vi "Dashboard Main.vi"() -> ()   [LabVIEW 2015]
uses:
  <vilib>/Rock Robotics/WPI/DriverStation/WPI_DriverStationRobotMode2.ctl
  <vilib>/event_ctls.llb/eventvkey.ctl
  <vilib>/Rock Robotics/WPI/Dashboard/WPI_DashboardLogging Global.vi
  <vilib>/Rock Robotics/Network Tables/NT Read Numeric Array.vi
  <vilib>/Rock Robotics/Network Tables/SD Read Number.vi
  <vilib>/Rock Robotics/Network Tables/SD Write Number.vi
  <vilib>/Rock Robotics/Network Tables/SD Write Boolean.vi
  <vilib>/Rock Robotics/Network Tables/SD Read Boolean.vi
  <vilib>/Rock Robotics/Network Tables/NT Write Boolean.vi
  <vilib>/Utility/config.llb/Write Key (String).vi
  <vilib>/Utility/config.llb/Write Key (I32).vi
  <vilib>/Utility/config.llb/NI_LVConfig.lvlib
panel:
  out "x = 0?":bool[](array[boolean])
  in  "TCP":refnum<k5>
  out "Camera IP":string
  out "Image Message":string="Timeout in Camera Communications"
  in  "Dashboard Tab":T1(tab)
  in  "Force Aim":bool
  in  "Enable Shooter":bool=TRUE
  in  "Intake to top?":bool=TRUE
  in  "Straight Forward":bool
  in  "Camera Settings":T2={"Frame Rate"=30, "Compression"=30, "Size"=1} {"Frame Rate" scale=1.0..30.0; "Size" items=["640x480", "320x240", "160x120"]}
  out "MotorChart R":cluster{"Numeric":dbl, "Numeric":dbl}(graph)
  out "MotorChart L":T3(graph)
  out "MotorSliders R":cluster{"MotorSlide1":dbl, "MotorSlide2":dbl} {"MotorSlide2" scale=-1.0..1.0 scale format="%#_2e"; "MotorSlide1" scale=-1.0..1.0 scale format="%#_2e"}
  out "MotorSliders L":T4 {"MotorSlide4 2" scale=0.0..14.0 scale format="%#_2e"; "MotorSlide2" scale=-1.0..1.0 scale format="%#_2e"; "MotorSlide1" scale=-1.0..1.0 scale format="%#_2e"}
  out "Yaw":dbl(knob) scale=180.0..-180.0
  out "JS1 Z":dbl(slide) scale=-1.0..1.0 scale format="%#_2e"
  out "JS1 Graph":cluster{"X":dbl, "Y":dbl}[](graph)
  out "JS1 Buttons":T5
  out "JS2 Z":dbl(slide) scale=-1.0..1.0 scale format="%#_2e"
  out "JS2 Graph":cluster{"X":dbl, "Y":dbl}[](graph)
  out "JS2 Buttons":T5
  out "Mode":T6(ring)=enum."Auto Disabled"
  in  "DB Camera Config":bool
  out "fps":dbl format="%#.1g"
  out "Mbps":dbl format="%#.1g"
  out "Mbps 2":bool
  out "Goal Detected":bool
  out "Ball Detected":bool
  in  "Start with Ball?":bool
  in  "Drive speed (0-1)":dbl
  in  "In. to Drive":dbl
  in  "Start Position":T7(ring)
  in  "Drive Back?":bool
  in  "Auto Mode":T8(ring)
  in  "Turn Around?":bool
  out "CAN Errors":T9(graph)
  out "Drive":T9(graph)
  out "Current":T9(graph)
  out "Drive Throttle":T9(graph)
  out "?":T10(graph)
  out "?":T9(graph)
  out "?":T10(graph)
  out "?":T10(graph)
  out "?":T9(graph)
  out "?":T10(graph)
  out "?":T9(graph)
  out "?":T9(graph)
  in  "Test Slider":dbl(slide) scale=0.0..100.0 scale format="%#_3g"
  in  "On/Off":bool caption="Solenoid"
  in  "Test Name":u16(ring) items=["Select the test to run...", "Example Test", "-------------------------------", "List of tests is built in robot code.", "Replace with your own automated tests."]
  in  "Test Tree":string(tree)
  in  "Motor":cluster{"Value":dbl, "Enable":bool} {"Value" scale=-1.0..1.0 scale format="%#_3g"}
  out "Progress":T11 {"Test Progress" scale=0.0..100.0}
  in  "Rev/Fwd":cluster{"Forward":bool, "Reverse":bool}
  in  "Test Ring":u16(ring) items=["Monochrome", "Color"]
  in  "Vision":u16(ring) items=["Camera Off", "USB Camera SW", "USB Camera HW", "IP Camera"]
  in  "Rec Mode":enum32{"Stop", "Record", "Playback"}(radio)
  in  "Listbox":i32(listbox)
  out "Tree":string(tree)
  out "Camera Image":T12(plugin-control)
  out "Turn Around?":bool
  # "Left"
  # "Front"
  # "Right"
  # "Battery"
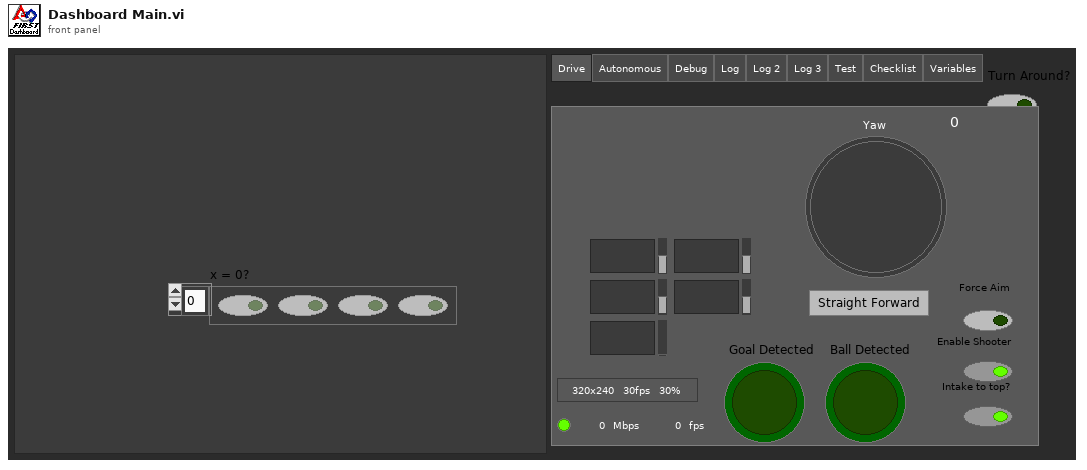
[diagram p1: front panel]
types:
  T1 = enum32{"Drive", "Autonomous", "Debug", "Log", "Log 2", "Log 3", "Test", "Checklist", "Variables"}
  T2 = cluster{"Frame Rate":i32, "Compression":i32, "Size":u16}
  T3 = cluster{"Numeric":dbl, "Numeric":dbl, "Battery V":dbl}
  T4 = cluster{"MotorSlide1":dbl, "MotorSlide2":dbl, "MotorSlide4 2":dbl}
  T5 = cluster{bool, bool, bool, bool, bool, bool, bool, bool, bool, bool, bool, bool}
  T6 = enum8{"Tele-Op Disabled", "Tele-Op Enabled", "Auto Disabled", "Auto Enabled", "Test Disabled", "Test Enabled", "Disconnected", "No Code", "E-Stop"}
  T7 = enum16{"Defense 1", "Defense 2", "Defense 3", "Defense 4", "Defense 5"}
  T8 = enum16{"Nothing", "Nothing+aim", "Drive", "Drive+aim", "Shoot +Drive", "Low Goal +Drive"}
  T9 = cluster{"Numeric Array[0]":dbl, "Numeric Array[1]":dbl, "Numeric Array[2]":dbl, "Numeric Array[3]":dbl, "Numeric Array[4]":dbl, "Numeric Array[5]":dbl, "Numeric Array[6]":dbl, "Numeric Array[7]":dbl, "Numeric Array[8]":dbl, "Numeric Array[9]":dbl}
  T10 = cluster{"Numeric Array[0]":dbl, "Numeric Array[1]":dbl, "Numeric Array[2]":dbl, "Numeric Array[3]":dbl, "Numeric Array[4]":dbl, "Numeric Array[5]":dbl, "Numeric Array[6]":dbl, "Numeric Array[7]":dbl, "Numeric Array[8]":dbl}
  T11 = cluster{"Test Progress":u8, "Test Progress Text":string}
  T12 = typedef "IMAQ Image.ctl" = refnum<image>
  T13 = enum32{"Drive", "Basic", "Custom", "Test", "Checklist", "Variables"}
  T14 = typedef "Image Type" = u32
  T15 = typedef "NI_LVConfig.lvlib/Config Data RefNum.ctl" = refnum<k1>
  T16 = typedef "WPI_DriverStationRobotMode2.ctl" = enum16{"Autonomous Disabled", "Autonomous Enabled", "Teleop Disabled", "Teleop Enabled", "Disconnected", "Finish", "Test Disabled", "Test Enabled", "Emergency Stopped"}
  T17 = cluster{"Camera Image":refnum<vi>, "Dashboard Tab":refnum<vi>, "Turn Around?":refnum<vi>, "Vision":refnum<vi>, "Rec Mode":refnum<vi>, "Test Slider":refnum<vi>, "On/Off ":refnum<vi>, "Test Ring":refnum<vi>, "Rev/Fwd":refnum<vi>, "Test Name":refnum<vi>, "Motor":refnum<vi>, "Progress":refnum<vi>, "Listbox":refnum<vi>, "Tree":refnum<vi>, "Test Tree":refnum<vi>}
  T18 = cluster{"Error Strings":string, "Disable Counts":cluster{u16, u16}, "Rail Faults":cluster{u16, u16, u16}, "Robot IP":string, "DB Mode":u8, "Event Info":cluster{"Name":string, "Type":u8, "Number":u16, "Replay":u8}, "Camera Addr":string}
  T19 = cluster{"Storage":cluster{"Disk Free":u64, "RAM Block":u32, "RAM free":u32}, "CPU Utilization":cluster{"CPU % ISR":sgl, "CPU % Time Crit":sgl, "CPU % Timed Str":sgl, "CPU % High":sgl, "CPU % Above":sgl, "CPU % Normal":sgl, "CPU % Low":sgl}, "CAN":cluster{"% Bus Utilization":sgl, "Bus Off Cnt":u32, "TX_FIFO Full Cnt":u32, "Receive Error Cnt":u8, "Transmit Error Cnt":u8}, "HID":cluster{"HID Outputs":u32, "Rumble Low":u16, "Rumble High":u16}[]}
  T20 = cluster{"Status bits":cluster{"Test Mode":bool, "Autonomous":bool, "Enabled":bool, "Code Start":bool, "Brownout":bool, "Reserved 2":bool, "Reserved 3":bool, "E-Stop":bool}, "Code Trace":cluster{"Disabled":bool, "TeleOp":bool, "Auto":bool, "Test":bool}, "Controller Type":enum16{"unknown", "cRIO", "roboRio"}, "Code?":enum16{"unknown", "noCode", "code"}, "Battery V":dbl}
  T21 = cluster{"Control Bits":cluster{"TestMode":bool, "Autonomous":bool, "Enabled":bool, "FMS Present":bool, bool, bool, bool, "E-Stop":bool}, "Team Station ":u8, "Countdown":sgl, "Joystick Values":cluster{"Axes":dbl[], "Buttons":bool[], "POVs":i16[]}[]}
  T22 = cluster{"Axes":dbl[], "Buttons":bool[], "POVs":i16[]}[]
  T23 = cluster{"Axes":dbl[], "Buttons":bool[], "POVs":i16[]}
  T24 = cluster{"Buttons[0]":bool, "Buttons[1]":bool, "Buttons[2]":bool, "Buttons[3]":bool, "Buttons[4]":bool, "Buttons[5]":bool, "Buttons[6]":bool, "Buttons[7]":bool, "Buttons[8]":bool, "Buttons[9]":bool, "Buttons[10]":bool, "Buttons[11]":bool}
  T25 = cluster{"[0]":dbl, "[1]":dbl, "[2]":dbl, "[3]":dbl, "[4]":dbl, "[5]":dbl, "[6]":dbl, "[7]":dbl, "[8]":dbl, "[9]":dbl}
  T26 = cluster{"Operation":enum16{"Update", "Clear"}, "Color Box":u32}[]
  T27 = typedef "eventvkey.ctl" = enum16{"ASCII", "Enter", "Return", "Shift", "Ctrl", "Alt", "Cmd", "Opt", "Caps", "NumLock", "Clear", "Break", "Up", "Down", "Left", "Right", "Insert", "Delete", "Home", "End", "PageUp", "PageDown", "Escape", "Help", "Pause", "ScrollLock", "F1", "F2", "F3", "F4", "F5", "F6", "F7", "F8", "F9", "F10", "F11", "F12", "F13", "F14", "F15", "F16", "F17", "F18", "F19", "F20", "F21", "F22", "F23", "F24", "Play", "VolumeUp", "VolumeDown", "Mute", "Two Byte Char"}
  T28 = cluster{"Image Size":bool, "Image Type":bool, "Pixel Value":bool, "ROI Information":bool, "Zoom Factor":bool}
  T29 = enum8{"Enabled", "Disabled", "Disabled and Grayed Out"}
  T30 = cluster{"Operation":enum16{"Update", "Clear"}, "Color Box":u32}
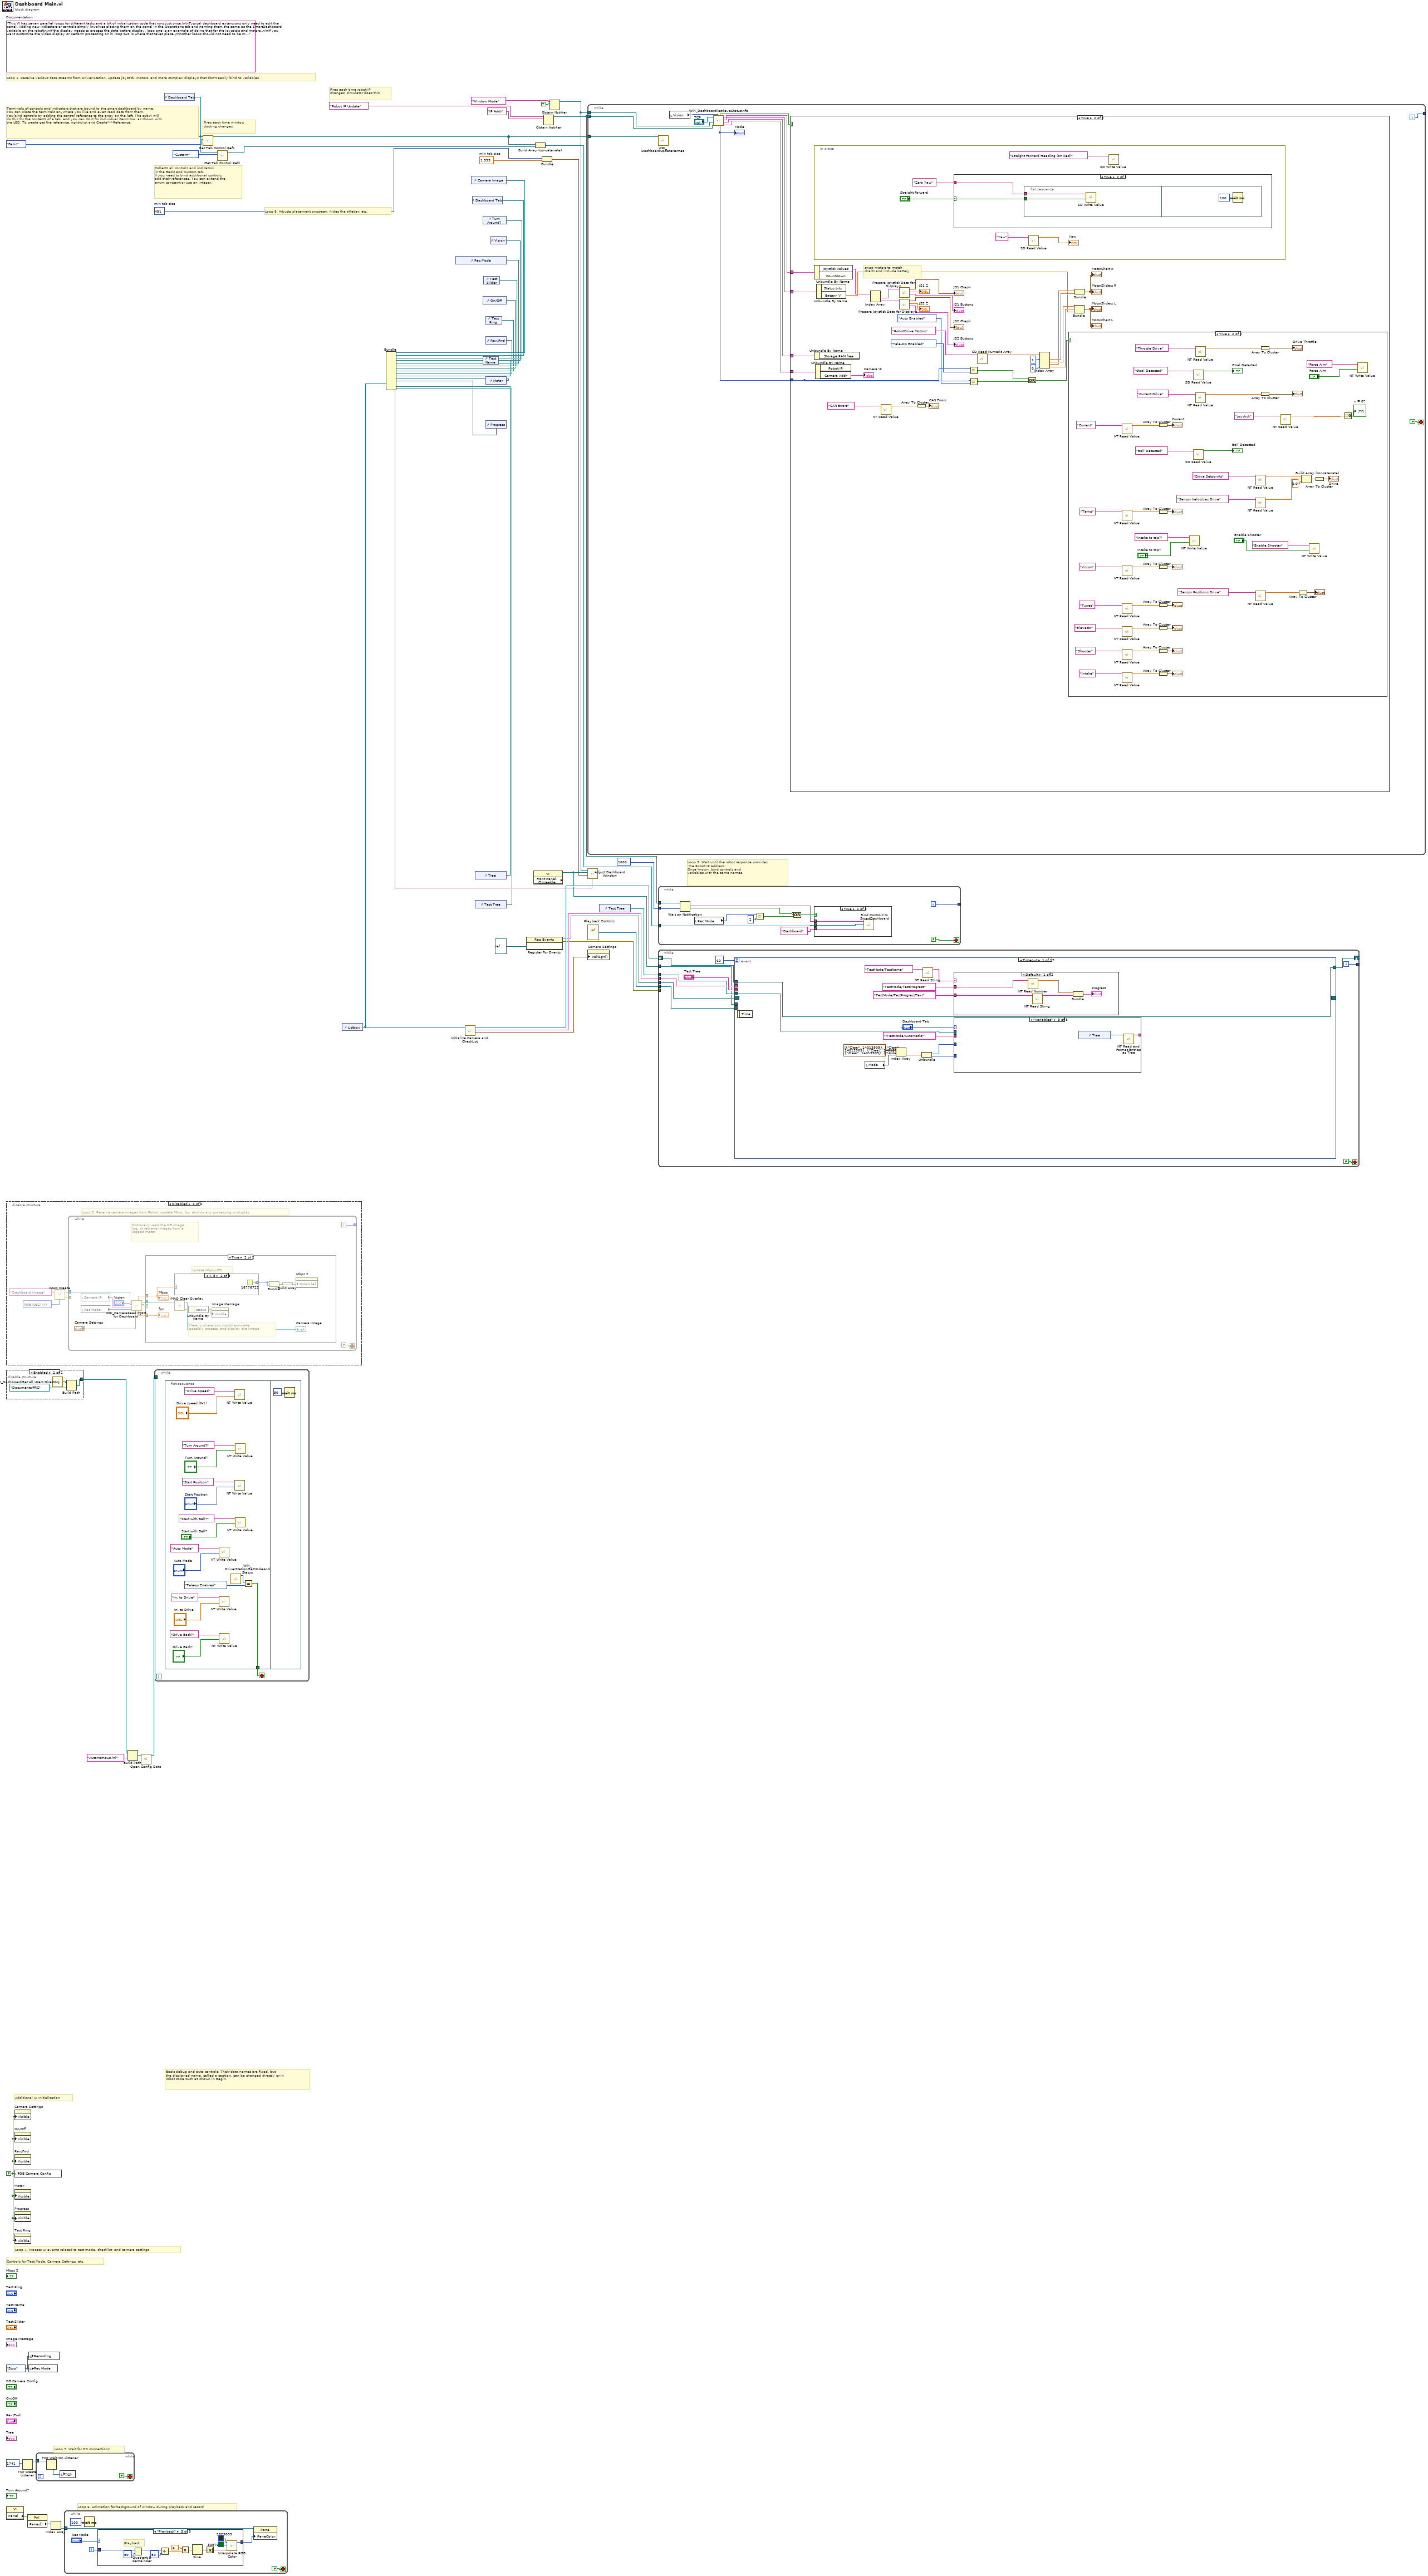
[diagram p0: block diagram]
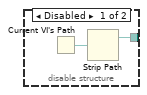
[diagram p2: hidden frame]
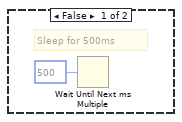
[diagram p3: hidden frame]
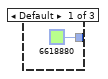
[diagram p4: hidden frame]
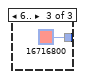
[diagram p5: hidden frame]
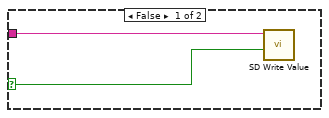
[diagram p9: hidden frame]
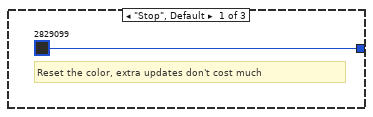
[diagram p10: hidden frame]
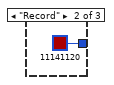
[diagram p11: hidden frame]
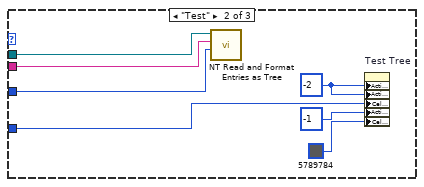
[diagram p14: hidden frame]
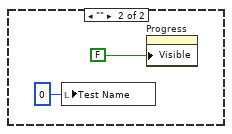
[diagram p15: hidden frame]
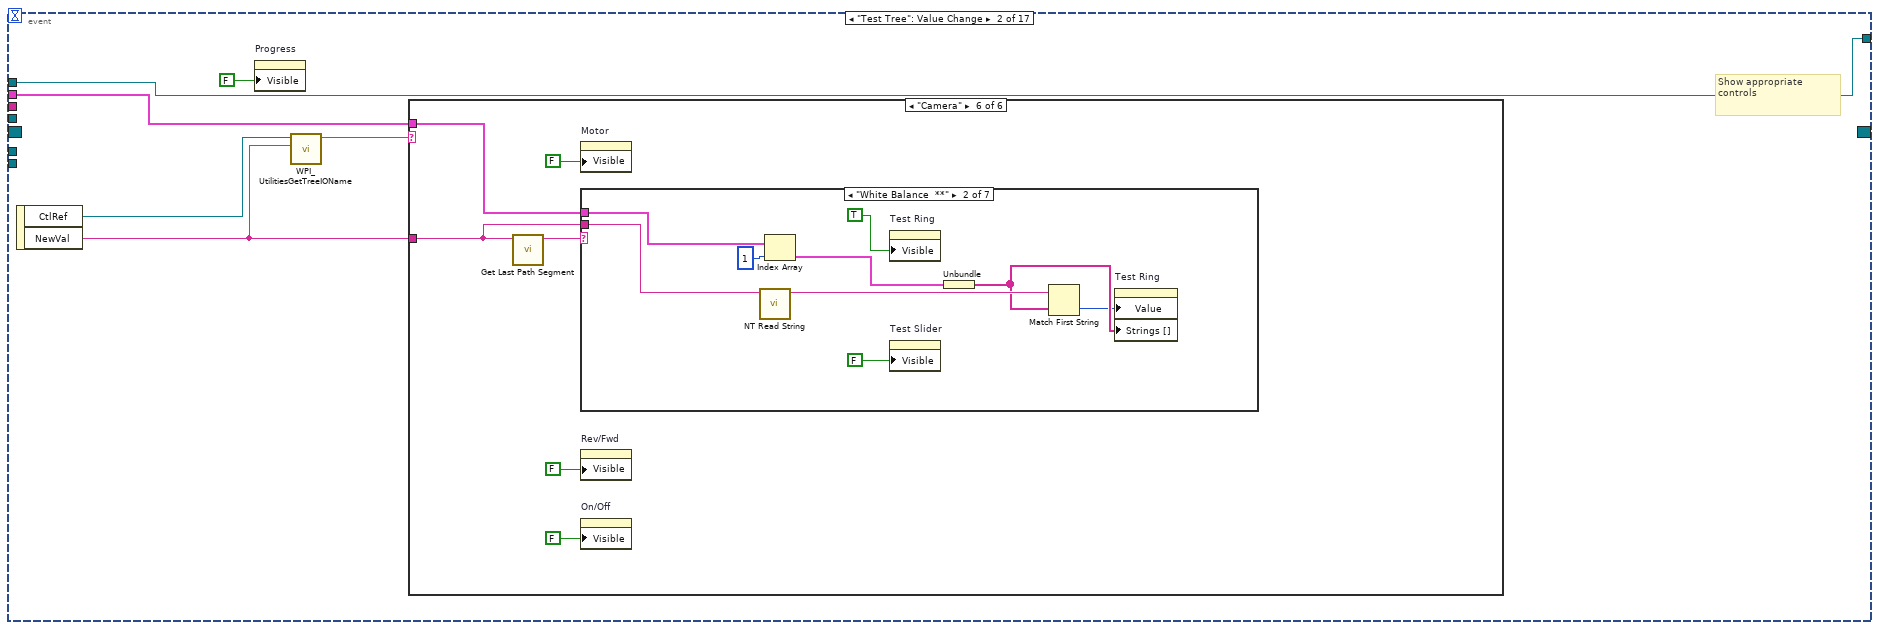
[diagram p16: hidden frame]
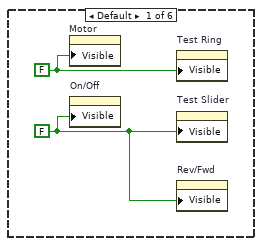
[diagram p17: hidden frame]
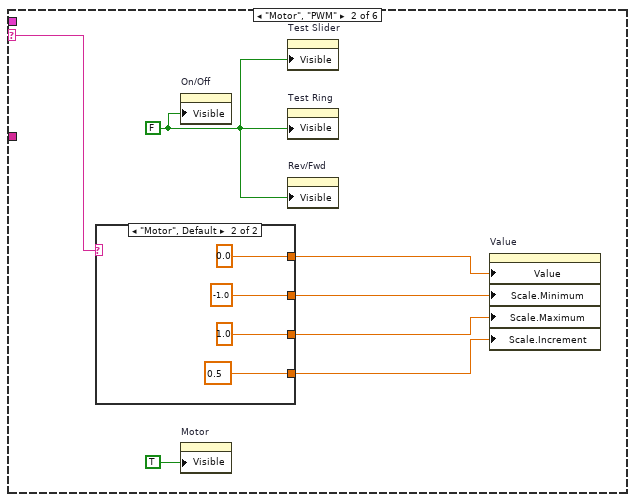
[diagram p18: hidden frame]
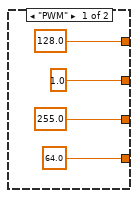
[diagram p19: hidden frame]
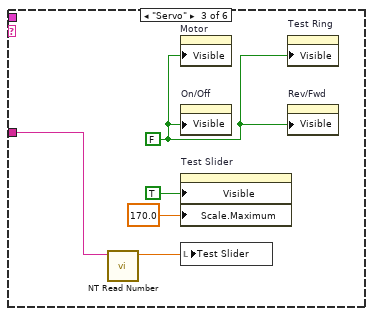
[diagram p20: hidden frame]
diagram:
  w28 = 491  # min tab size
  w27 = 1.333  # min tab size
  w36 = enum32{"Stop", "Record", "Playback"}."Stop" ("Rec Mode")
  w11 = FALSE ("Visible")
  (unwired) "This VI has seven parallel loops for different tasks and a bit of initialization code that runs just once.\n\nTypical dashboard extensions only need to edit the panel. Adding new indicators or controls simply involves placing them on the panel in the Operations tab and naming them the same as the SmartDashboard variable on the robot\n\nIf the display needs to process the data before display, loop one is an example of doing that for the joysticks and motors.\n\nIf you want customize the video display or perform processing on it, loop two is where that takes place.\n\nOther loops should not need to be modified. They are pretty standard, and document the task they perform."  # Documentation
  # "Loop 7. Wait for DS connections"
  # "Basic debug and auto controls: Their data names are fixed, but\nthe displayed name, called a caption, can be changed directly or in\nrobot code such as shown in Begin."
  # "Controls for Test Mode, Camera Settings, etc."
  # "Additional UI Initialization"
  # "Loop 6. Animation for background of window during playback and record"
  # "Fires each time robot IP\nchanges, simulator does this"
  # "Fires each time window\ndocking changes."
  # "Collects all controls and indicators\nin the Basic and Custom tab.\nIf you need to bind additional controls,\nadd their references. You can extend the\nenum constant or use an integer."
  # "Loop 4. Process UI events related to test mode, checklist, and camera settings"
  # "Terminals of controls and indicators that are bound to the smart dashboard by name.\nYou can place the terminals anywhere you like and even read data from them.\nYou bind controls by adding the control reference to the array on the left. The subVI will\ndo this for the contents of a tab, and you can do it for individual items too, as shown with\nthe LED. To create get the reference, right-click and Create>>Reference."
  # "Loop 3. Wait until the robot response provides\n the Robot IP address.\nOnce known, bind controls and\nvariables with the same names."
  # "Loop 5. Adjusts placement onscreen, hides the titlebar, etc."
  # "Loop 1. Receive various data streams from Driver Station, update joystick, motors, and more complex displays that don't easily bind to variables."
  n1 = disable-structure shown="Disabled" {
    frame Disabled {
      w56 = T14 4 items=["Grayscale (U8)", "Grayscale (I16)", "Grayscale (SGL)", "Complex (CSG)", "RGB (U32)", "HSL (U32)", "RGB (U64)"] ("Image Type")
      # "Loop 2. Receive camera images from Robot, update Mbps, fps, and do any processing or display"
      n2 = call "IMAQ Create"("Image Name"="Dashboard Image", "Image Type"=w56) -> ("New Image"=w54:T12, "error out"=w53:errorcluster)  [unwired: 2 in, 1 out]
      n3 = while {
        tunnel: w54 -> [w65]
        tunnel: w53 -> [_]
        tunnel: [w66] -> _
        i -> [w66]
        stop <- FALSE stop-if-true
        # "Optionally read the DB image,\nlog, or retrieve images from a\nlogged match"
        n4 = local read "Camera IP"() -> (w57:string)
        n5 = local read "Rec Mode"() -> (w59:enum32{"Stop", "Record", "Playback"})
        n6 = call <vilib>:"WPI_CameraRead MJPG for Dashboard.vi"("Camera Settings"="Camera Settings", "Rec Mode"=w59, "Camera IP"=w57, "Camera Mode"="Vision", "Refnum in"=w65) -> ("Active"=w63:bool, "Refnum out"=w64:T12, "FPS"=w62:dbl, "Bandwidth (Mbps)"=w61:dbl)  [unwired: 3 in]
        n7 = case shown="True" w63 {
          tunnel: w64 -> [_ w72]
          tunnel: w61 -> [_ w71]
          tunnel: w62 -> [_ w69]
          frame False {
            # "Sleep for 500ms"
            n8 = Wait Until Next ms Multiple(millisecond multiple=u32 500) -> ()  [unwired: 1 out]
          }
          frame True {
            # "Here is where you would annotate,\npossibly process, and display the image"
            # "Update Mbps LED"
            n9 = case shown="4, 5" w71 {
              tunnel: [u32 6618880 ("Color Box") u32 16776722 ("Color Box") u32 16716800 ("Color Box")] -> w73
              frame Default {
              }
              frame 4, 5 {
              }
              frame 6.. {
              }
            }
            n10 = call "IMAQ Clear Overlay"("Image"=w72) -> ("error out"=w76:errorcluster, "Image Out"=→"Camera Image":T12)  [unwired: 2 in, 7 out]
            n11 = Unbundle By Name(w76) -> ("status"=w77:bool)
            n12 = property on="Image Message" class="Str"("Visible"=w77) -> ()  [unwired: 2 in, 2 out]
            n13 = Bundle("Color Box"=w73, "Color Box"=w73) -> (w75:cluster{"Color Box":u32, "Color Box":u32})  [unwired: 1 out]
            n14 = Build Array(w75) -> (w74:cluster{"Color Box":u32, "Color Box":u32}[])
            n15 = property on="Mbps 2" class="Bool (strict)"("Colors [4]"=w74) -> ()  [unwired: 2 in, 2 out]
            "Mbps" <- w71
            "fps" <- w69
          }
        }
      }
    }
    frame Enabled {
    }
  }
  n16 = disable-structure shown="Enabled" {
    disable-tunnel: [w82 w85] -> w2
    frame Disabled {
      n17 = Current VI's Path() -> (path=w81:path)
      n18 = Strip Path(path=w81) -> (stripped path=w82:path)  [unwired: 1 out]
    }
    frame Enabled {
      n19 = call <vilib>:"WPI_DashboardGet All Users Directory.vi"() -> ("All User Path"=w83:path)
      n20 = Build Path(base path=w83, name or relative path=path "Documents/FRC" ("path")) -> (appended path=w85:path)
    }
  }
  n21 = property class="VI"() -> ("Panel"=w43:refnum<vi>)  [unwired: 2 in, 2 out]
  n22 = property on="Camera Settings" class="Clust (strict)"("Visible"=w11) -> ()  [unwired: 2 in, 2 out]
  n23 = property on="On/Off" class="Bool (strict)"("Visible"=w11) -> ()  [unwired: 2 in, 2 out]
  n24 = property on="Rev/Fwd" class="Clust (strict)"("Visible"=w11) -> ()  [unwired: 2 in, 2 out]
  n25 = local write "DB Camera Config"(w11) -> ()
  n26 = property on="Motor" class="Clust (strict)"("Visible"=w11) -> ()  [unwired: 2 in, 2 out]
  n27 = property on="Progress" class="Clust (strict)"("Visible"=w11) -> ()  [unwired: 2 in, 2 out]
  n28 = property on="Test Ring" class="Ring (strict)"("Visible"=w11) -> ()  [unwired: 2 in, 2 out]
  n29 = TCP Create Listener(10:u16 1741 ("timeout ms (25000)")) -> (3:w6:refnum<k5>)  [unwired: 4 in, 2 out]
  n30 = property class="Pnl"(reference=w43) -> ("Panes[]"=w44:refnum<vi>[])  [unwired: 1 in, 2 out]
  n31 = global write "WPI_DashboardLogging Global.vi" "Recording"(w36) -> ()
  n32 = local write "Rec Mode"(w36) -> ()
  n33 = while {
    tunnel: w6 -> [w87]
    stop <- FALSE stop-if-true
    n34 = TCP Wait On Listener(11:w87) -> (4:w86:refnum<k5>)  [unwired: 3 in, 4 out]
    n35 = local write "TCP"(w86) -> ()
  }
  n36 = Index Array(array=w44) -> (element=w42:refnum<vi>)  [unwired: 1 in]
  n37 = while {
    tunnel: w42 -> [w90]
    i -> [w93]
    stop <- FALSE stop-if-true
    n38 = Wait (ms)(milliseconds to wait=u32 100) -> ()  [unwired: 1 out]
    n39 = case shown="\"Playback\"" "Rec Mode" {
      tunnel: w93 -> [_ _ w108]
      tunnel: [u32 2829099 ("Base Color") u32 11141120 ("Target Color") w97] -> w89
      frame "Stop", Default {
        # "Reset the color, extra updates don't cost much"
      }
      frame "Record" {
      }
      frame "Playback" {
        # "Playback"
        n40 = Quotient & Remainder(x=w108, y=u32 50 ("milliseconds to wait")) -> (x-y*floor(x/y)=w104:u32)  [unwired: 1 out]
        n41 = Divide(x=w104, y=u32 50 ("milliseconds to wait")) -> (x/y=w101:dbl)
        n42 = Multiply(x=6.283185307179586, y=w101) -> (x*y=w106:dbl)
        n43 = Sine(x=w106) -> (sin(x)=w105:dbl)
        n44 = Absolute Value(x=w105) -> (abs(x)=w98:dbl)
        n45 = call "Interpolate RGB Color.vi"("Proportion"=w98, "Target Color"=u32 30976, "Base Color"=u32 2829099) -> ("Result Color"=w97:u32)  [unwired: 8 in]
      }
    }
    n46 = property class="Pane"(reference=w90, "PaneColor"=w89) -> ()  [unwired: 1 in, 2 out]
  }
  n47 = Build Path(base path=w2, name or relative path="Autonomous.ini") -> (appended path=w5:path)
  n48 = call <vilib>:"Open Config Data.vi"("configuration file path"=w5) -> ("refnum"=w3:T15)  [unwired: 8 in, 2 out]
  n49 = while {
    tunnel: w3 -> [_]
    stop <- w109 stop-if-true
    n50 = flat-sequence {
      tunnel: [w124] -> w109
      frame #0 {
        n51 = call-poly <vilib>:"NT Write Value.vi"("Numeric"="Auto Mode", "Name"="Auto Mode") -> ()  [unwired: 9 in, 1 out]
        n52 = call-poly <vilib>:"NT Write Value.vi"("Numeric"="In. to Drive", "Name"="In. to Drive") -> ()  [unwired: 9 in, 1 out]
        n53 = call-poly <vilib>:"NT Write Value.vi"("Boolean"="Drive Back?", "Name"="Drive Back?") -> ()  [unwired: 9 in, 1 out]
        n54 = call <vilib>:"WPI_DriverStationGetModeAndStatus.vi"() -> ("Robot Mode"=w126:T16)  [unwired: 10 in, 1 out]
        n55 = call-poly <vilib>:"NT Write Value.vi"("Numeric"="Drive speed (0-1)", "Name"="Drive Speed") -> ()  [unwired: 9 in, 1 out]
        n56 = call-poly <vilib>:"NT Write Value.vi"("Numeric"="Start Position", "Name"="Start Position") -> ()  [unwired: 9 in, 1 out]
        n57 = call-poly <vilib>:"NT Write Value.vi"("Boolean"="Turn Around?", "Name"="Turn Around?") -> ()  [unwired: 9 in, 1 out]
        n58 = call-poly <vilib>:"NT Write Value.vi"("Boolean"="Start with Ball?", "Name"="Start with Ball?") -> ()  [unwired: 9 in, 1 out]
        n59 = Equal?(x=w126, y=WPI_DriverStationRobotMode2."Teleop Enabled") -> (x = y?=w124:bool)
      }
      frame #1 {
        n60 = Wait (ms)(milliseconds to wait=50) -> ()  [unwired: 1 out]
      }
    }
  }
  n61 = control-ref of="Dashboard Tab"() -> (w34:refnum<vi>)
  n62 = call <vilib>:"Get Tab Control Refs.vi"("Page Index"=T13."Basic" ("Dashboard Tab"), "TabControl in"=w34) -> ("ControlsOnPage"=w9:refnum<vi>[])  [unwired: 9 in]
  n63 = call <vilib>:"Get Tab Control Refs.vi"("Page Index"=T13."Custom" ("Dashboard Tab"), "TabControl in"=w34) -> ("ControlsOnPage"=w33:refnum<vi>[])  [unwired: 9 in]
  n64 = control-ref of="Listbox"() -> (w1:refnum<vi>)
  n65 = control-ref of="Rec Mode"() -> (w17:refnum<vi>)
  n66 = call "Initialize Camera and CheckList.vi"("ListBox in"=w1) -> ("Cluster"=w47:cluster{"value":i32, "value":i32, "index":i32}, "Array"=w48:cluster{string[]}[], "File Refnum"=w46:T15)  [unwired: 8 in]
  n67 = control-ref of="Camera Image"() -> (w31:refnum<vi>)
  n68 = control-ref of="Dashboard Tab"() -> (w30:refnum<vi>)
  n69 = control-ref of="Tree"() -> (w21:refnum<vi>)
  n70 = control-ref of="Test Tree"() -> (w20:refnum<vi>)
  n71 = control-ref of="Turn Around?"() -> (w25:refnum<vi>)
  n72 = control-ref of="On/Off"() -> (w15:refnum<vi>)
  n73 = control-ref of="Test Name"() -> (w19:refnum<vi>)
  n74 = control-ref of="Test Slider"() -> (w16:refnum<vi>)
  n75 = control-ref of="Test Ring"() -> (w14:refnum<vi>)
  n76 = control-ref of="Rev/Fwd"() -> (w13:refnum<vi>)
  n77 = control-ref of="Motor"() -> (w18:refnum<vi>)
  n78 = control-ref of="Progress"() -> (w12:refnum<vi>)
  n79 = control-ref of="Vision"() -> (w29:refnum<vi>)
  n80 = Bundle("Camera Image"=w31, "Dashboard Tab"=w30, "Turn Around?"=w25, "Vision"=w29, "Rec Mode"=w17, "Test Slider"=w16, "On/Off"=w15, "Test Ring"=w14, "Rev/Fwd"=w13, "Test Name"=w19, "Motor"=w18, "Progress"=w12, "Listbox"=w1, "Tree"=w21, "Test Tree"=w20) -> (w22:T17)  [unwired: 1 in]
  n81 = register-events(refnum<vi> refnum) -> (reference out=w40:refnum<event-registration>, error out=w39:errorcluster)  [unwired: 2 in]
  n82 = property class="VI" props=["Front Panel.Closeable"]() -> (reference out=w35:refnum<vi>)  [unwired: 2 in, 2 out]
  n83 = Build Array (concatenate)(w9, w33) -> (w32:refnum<vi>[])
  n84 = Bundle("min tab size"=w28, "min tab size"=w27) -> (w26:cluster{"min tab size":i32, "min tab size":dbl})  [unwired: 1 in]
  n85 = Obtain Notifier(name (unnamed)="Robot IP Update", notification data type="IP Addr" ("name (unnamed)")) -> (notifier out=w10:refnum<notifier>)  [unwired: 2 in, 2 out]
  n86 = Obtain Notifier(name (unnamed)="Window Mode", notification data type=TRUE) -> (notifier out=w8:refnum<notifier>)  [unwired: 2 in, 2 out]
  n87 = while {
    tunnel: [w139] -> _
    tunnel: w10 -> [w133]
    tunnel: w9 -> [w132]
    tunnel: w8 -> [w128]
    i -> [w139]
    stop <- FALSE stop-if-true
    n88 = call <vilib>:"WPI_DashboardUpdateNames.vi"("Controls on Tab"=w132) -> ()  [unwired: 11 in]
    n89 = local read "Vision"() -> (w130:u16)
    n90 = call <vilib>:"WPI_DashboardRetrieveStatusInfo.vi"("Vision"=w130, "Binding Refnum"=w133, "Window Mode Notifier"=w128, "TCP Cnx"="TCP") -> ("Power and Errors"=w134:T18, "Robot Metrics"=w137:T19, "Status Info"=w138:T20, "Control Info"=w135:T21, "Robot Mode"=w131:T6, "Process?"=w136:bool)  [unwired: 2 in]
    "Mode" <- w131
    n91 = case shown="True" w136 {
      tunnel: w138 -> [_ w174]
      tunnel: w137 -> [_ w173]
      tunnel: w135 -> [_ w172]
      tunnel: w134 -> [_ w171]
      tunnel: w131 -> [_ w145]
      frame False {
      }
      frame True {
        # "swap motors to match\ncharts and include battery"
        n92 = in-place {
          n93 = case shown="True" "Straight Forward" {
            selector: "Straight Forward" -> [w230 w232]
            tunnel: "Zero Yaw" ("Name") -> [w231 w233]
            frame False {
              n94 = call-poly <vilib>:"SD Write Value.vi"("Boolean"=w230, "Name"=w231) -> ()  [unwired: 8 in, 2 out]
            }
            frame True {
              n95 = flat-sequence {
                tunnel: w233 -> [w235]
                tunnel: w232 -> [w234]
                frame #0 {
                  n96 = call-poly <vilib>:"SD Write Value.vi"("Boolean"=w234, "Name"=w235) -> ()  [unwired: 8 in, 2 out]
                }
                frame #1 {
                  n97 = Wait (ms)(milliseconds to wait=u32 100) -> ()  [unwired: 1 out]
                }
              }
            }
          }
          n98 = call-poly <vilib>:"SD Read Value.vi"("Name"="Yaw") -> ("Numeric"=→"Yaw":dbl)  [unwired: 8 in, 2 out]
          n99 = call-poly <vilib>:"SD Write Value.vi"("Name"="Straight Forward Heading (on Red)") -> ()  [unwired: 9 in, 2 out]
        }
        n100 = Unbundle By Name(w172) -> ("Joystick Values"=w159:T22)  [unwired: 1 out]
        n101 = Unbundle By Name(w173) -> ()  [unwired: 1 out]
        n102 = Unbundle By Name(w171) -> ("Camera Addr"=→"Camera IP":string)  [unwired: 1 out]
        n103 = Unbundle By Name(w174) -> ("Battery V"=w160:dbl)  [unwired: 1 out]
        n104 = Index Array(array=w159) -> (element #1=w158:T23, element #2=w153:T23)  [unwired: 2 in]
        n105 = call-poly <vilib>:"NT Read Value.vi"("Name"="CAN Errors") -> ("Numeric Array"=w142:dbl[])  [unwired: 9 in, 1 out]
        n106 = call "Prepare Joystick Data for Displays.vi"("Joystick Values"=w158) -> ("Buttons"=→"JS1 Buttons":T24, "Z Axis"=→"JS1 Z":dbl, "Cartesian Data"=→"JS1 Graph":cluster{"X axis":dbl, "X axis":dbl}[])  [unwired: 8 in]
        n107 = call "Prepare Joystick Data for Displays.vi"("Joystick Values"=w153) -> ("Buttons"=→"JS2 Buttons":T24, "Z Axis"=→"JS2 Z":dbl, "Cartesian Data"=→"JS2 Graph":cluster{"X axis":dbl, "X axis":dbl}[])  [unwired: 8 in]
        n108 = Array To Cluster(array=w142) -> (cluster=→"CAN Errors":T9)
        n109 = Equal?(x=w145, y=T6."Tele-Op Enabled") -> (x = y?=w149:bool)
        n110 = Equal?(x=w145, y=T6."Auto Enabled") -> (x = y?=w146:bool)
        n111 = call <vilib>:"SD Read Numeric Array.vi"("Name"="RobotDrive Motors") -> ("Numeric Array"=w162:dbl[])  [unwired: 8 in, 2 out]
        n112 = Or(x=w149, y=w146) -> (x .or. y?=w147:bool)
        n113 = Index Array(array=w162, index #1=1, index #4=0) -> (element #1=w166:dbl, element #2=w167:dbl, element #3=w165:dbl, element #4=w170:dbl)  [unwired: 2 in]
        n114 = case shown="True" w147 {
          frame False {
          }
          frame True {
            n115 = call-poly <vilib>:"NT Read Value.vi"("Name"="Current") -> ("Numeric Array"=w210:dbl[])  [unwired: 9 in, 1 out]
            n116 = call-poly <vilib>:"NT Read Value.vi"("Name"="Temp") -> ("Numeric Array"=w191:dbl[])  [unwired: 9 in, 1 out]
            n117 = call-poly <vilib>:"NT Read Value.vi"("Name"="Vision") -> ("Numeric Array"=w199:dbl[])  [unwired: 9 in, 1 out]
            n118 = call-poly <vilib>:"NT Read Value.vi"("Name"="Turret") -> ("Numeric Array"=w189:dbl[])  [unwired: 9 in, 1 out]
            n119 = call-poly <vilib>:"NT Read Value.vi"("Name"="Elevator") -> ("Numeric Array"=w194:dbl[])  [unwired: 9 in, 1 out]
            n120 = call-poly <vilib>:"NT Read Value.vi"("Name"="Shooter") -> ("Numeric Array"=w193:dbl[])  [unwired: 9 in, 1 out]
            n121 = call-poly <vilib>:"NT Read Value.vi"("Name"="Intake") -> ("Numeric Array"=w202:dbl[])  [unwired: 9 in, 1 out]
            n122 = Array To Cluster(array=w210) -> (cluster=→"Current":T9)
            n123 = Array To Cluster(array=w191) -> (cluster=→"?":T10)
            n124 = Array To Cluster(array=w199) -> (cluster=→"?":T9)
            n125 = Array To Cluster(array=w189) -> (cluster=→"?":T9)
            n126 = Array To Cluster(array=w194) -> (cluster=→"?":T10)
            n127 = Array To Cluster(array=w193) -> (cluster=→"?":T10)
            n128 = Array To Cluster(array=w202) -> (cluster=→"?":T9)
            n129 = call-poly <vilib>:"NT Write Value.vi"("Boolean"="Intake to top?", "Name"="Intake to top?") -> ()  [unwired: 9 in, 1 out]
            n130 = call-poly <vilib>:"SD Read Value.vi"("Name"="Goal Detected") -> ("Boolean"=→"Goal Detected":bool)  [unwired: 8 in, 2 out]
            n131 = call-poly <vilib>:"SD Read Value.vi"("Name"="Ball Detected") -> ("Boolean"=→"Ball Detected":bool)  [unwired: 8 in, 2 out]
            n132 = call-poly <vilib>:"NT Read Value.vi"("Name"="Throttle Drive") -> ("Numeric Array"=w207:dbl[])  [unwired: 9 in, 1 out]
            n133 = call-poly <vilib>:"NT Read Value.vi"("Name"="Current Drive") -> ("Numeric Array"=w183:dbl[])  [unwired: 9 in, 1 out]
            n134 = call-poly <vilib>:"NT Read Value.vi"("Name"="Drive Setpoints") -> ("Numeric Array"=w215:dbl[])  [unwired: 9 in, 1 out]
            n135 = call-poly <vilib>:"NT Read Value.vi"("Name"="Sensor Velocities Drive") -> ("Numeric Array"=w214:dbl[])  [unwired: 9 in, 1 out]
            n136 = call-poly <vilib>:"NT Read Value.vi"("Name"="Sensor Positions Drive") -> ("Numeric Array"=w196:dbl[])  [unwired: 9 in, 1 out]
            n137 = Array To Cluster(array=w207) -> (cluster=→"Drive Throttle":T9)
            n138 = Array To Cluster(array=w183) -> (cluster=→"?":T10)
            n139 = call-poly <vilib>:"NT Read Value.vi"("Name"="joystick") -> ("Numeric Array"=w178:dbl[])  [unwired: 9 in, 1 out]
            n140 = Array To Cluster(array=w196) -> (cluster=→"?":T9)
            n141 = Build Array (concatenate)(w215, w214, 0.0) -> (w212:dbl[])
            n142 = call-poly <vilib>:"NT Write Value.vi"("Boolean"="Enable Shooter", "Name"="Enable Shooter") -> ()  [unwired: 9 in, 1 out]
            n143 = Array To Cluster(array=w212) -> (cluster=→"Drive":T25)
            n144 = Equal To 0?(x=w178) -> (x = 0?=→"x = 0?":bool[])
            n145 = call-poly <vilib>:"NT Write Value.vi"("Boolean"="Force Aim", "Name"="Force Aim") -> ()  [unwired: 9 in, 1 out]
          }
        }
        n146 = Bundle("Numeric"=w167, "Numeric"=w170, "Battery V"=w160) -> (→"MotorChart L" →"MotorSliders L":T3)  [unwired: 1 in]
        n147 = Bundle("Numeric"=w165, "Numeric"=w166) -> (→"MotorChart R" →"MotorSliders R":cluster{"Numeric":dbl, "Numeric":dbl})  [unwired: 1 in]
      }
    }
  }
  n148 = call "Adjust Dashboard Window.vi"("Sizing Refnums"=w22, "Size Constraints"=w26, "VI"=w35, "Notifier in"=w8) -> ()  [unwired: 8 in]
  n149 = vi-ref "Playback Controls.vi"() -> (w41:refnum<vi>)
  n150 = property on="Camera Settings" class="Clust (strict)"("Val(Sgnl)"=w47) -> ()  [unwired: 2 in, 2 out]
  n151 = control-ref of="Test Tree"() -> (w45:refnum<vi>)
  n152 = while {
    tunnel: w32 -> [w248]
    tunnel: w10 -> [w246]
    tunnel: [w244] -> _
    tunnel: u32 1000 ("milliseconds to wait") -> [w243]
    i -> [w244]
    stop <- FALSE stop-if-true
    n153 = Wait on Notification(notifier=w246, timeout in ms (-1)=w243) -> (notification=w245:string, timed out?=w241:bool)  [unwired: 2 in, 2 out]
    n154 = local read "Rec Mode"() -> (w239:enum32{"Stop", "Record", "Playback"})
    n155 = Equal?(x=w239, y=u16 2 ("Rec Mode")) -> (x = y?=w240:bool)
    n156 = Compound Arithmetic op=OR(invert w241, w240) -> (w242:bool)
    n157 = case shown="True" w242 {
      tunnel: w248 -> [_ w251]
      tunnel: w245 -> [_ w250]
      tunnel: "Dashboard" -> [_ w249]
      frame False {
      }
      frame True {
        n158 = call <vilib>:"Bind Controls to SmartDashboard.vi"("Client Name"=w249, "Bound Control Refs"=w251, "Server IP Address"=w250) -> ()  [unwired: 9 in]
      }
    }
  }
  n159 = while {
    tunnel: w48 -> [w259]
    shift-right: [w258] -> _
    shift-left: w46 -> [w257]
    tunnel: [w256] -> _
    tunnel: w45 -> [w255]
    tunnel: w41 -> [w254]
    tunnel: w40 -> [w253]
    tunnel: w39 -> [_]
    tunnel: w35 -> [w252]
    i -> [w256]
    stop <- FALSE stop-if-true
    n160 = event shown="[0] Timeout" {
      selector: w253 -> [_ _ _ _ _ _ _ _ _ _ _ _ _ _ _ _ _]
      dyn-events: [_ _ _ _ _ _ _ _ _ _ _ _ _ w497 _ _ _] -> _
      timeout: u32 60 ("milliseconds to wait") -> [_ _ _ _ _ _ _ _ _ _ _ _ _ _ _ _ _]
      tunnel: w255 -> [w271 _ _ _ _ _ _ _ _ _ _ _ _ _ _ _ _]
      tunnel: "Test Tree" -> [_ _ _ _ _ _ _ _ w466 w474 w476 w480 w488 _ _ _ _]
      tunnel: w259 -> [_ w293 _ _ _ _ w430 w460 _ _ _ _ _ _ _ _ _]
      tunnel: [w267 w292 w391 w396 w404 w416 w429 w453 w465 w472 w475 w479 w487 w499 w513 w514 w524] -> w258
      tunnel: w257 -> [w267 w292 w391 w396 w404 w416 w428 w453 w465 w472 w475 w479 w487 w499 w513 w514 w524]
      tunnel: w254 -> [_ _ _ _ _ _ _ _ _ _ _ _ _ w500 _ w517 _]
      tunnel: w252 -> [_ _ _ _ _ _ _ _ _ _ _ _ _ w495 _ _ _]
      event Timeout {
        n161 = event-data() -> ()  [unwired: 1 in, 1 out]
        n162 = local read "Mode"() -> (w270:T6)
        n163 = Index Array(array=T26 [{"Operation"=enum."Clear", "Color Box"=14013909}, {"Operation"=enum."Clear", "Color Box"=14013909}, {"Operation"=enum."Clear", "Color Box"=14013909}, {"Operation"=enum."Clear", "Color Box"=14013909}, {"Operation"=enum."Update", "Color Box"=14013909}, {"Operation"=enum."Update", "Color Box"=16777215}, {"Operation"=enum."Clear", "Color Box"=14013909}, {"Operation"=enum."Clear", "Color Box"=14013909}, {"Operation"=enum."Clear", "Color Box"=14013909}], index=w270) -> (element=w265:T30)
        n164 = Unbundle(w265) -> ("Operation"=w264:enum16{"Update", "Clear"}, "Color Box"=w263:u32)
        n165 = call <vilib>:"NT Read String.vi"("Name"="TestMode/TestName") -> ("String"=w274:string)  [unwired: 9 in, 1 out]
        n166 = case shown="Default" w274 {
          tunnel: "TestMode/TestProgress" ("Name") -> [w286 _]
          tunnel: "TestMode/TestProgressText" ("Name") -> [w285 _]
          frame Default {
            n167 = call <vilib>:"NT Read Number.vi"("Name"=w286) -> ("Numeric"=w287:dbl)  [unwired: 9 in, 1 out]
            n168 = call <vilib>:"NT Read String.vi"("Name"=w285) -> ("String"=w288:string)  [unwired: 9 in, 1 out]
            n169 = Bundle("Numeric"=w287, "String"=w288) -> (→"Progress":cluster{"Numeric":dbl, "String":string})  [unwired: 1 in]
          }
          frame "" {
            n170 = local write "Test Name"(u16 0) -> ()
            n171 = property on="Progress" class="Clust (strict)"("Visible"=FALSE) -> ()  [unwired: 2 in, 2 out]
          }
        }
        n172 = case shown="\"Variables\"" "Dashboard Tab" {
          tunnel: w271 -> [_ w282 _]
          tunnel: "/TestMode/Automatic/" ("Name Pattern") -> [_ w281 _]
          tunnel: w264 -> [_ w280 _]
          tunnel: [_ _ w284] -> _
          tunnel: w263 -> [_ w276 _]
          frame "Drive", Default {
          }
          frame "Test" {
            w279 = -2 ("Active Item:Row Number")
            n173 = call <vilib>:"NT Read and Format Entries as Tree.vi"("Operation"=w280, "Name Pattern"=w281, "Tree Refnum"=w282) -> ()  [unwired: 7 in, 2 out]
            n174 = property on="Test Tree" class="Tree (strict)"("Active Item Row Number"=w279, "ActiveColNum"=w279, "CellBG"=w276, "Active Item Row Number"=-1 ("Active Item:Row Number"), "CellBG"=u32 5789784 ("Color Box")) -> ()  [unwired: 2 in, 2 out]
          }
          frame "Variables" {
            n175 = control-ref of="Tree"() -> (w283:refnum<vi>)
            n176 = call <vilib>:"NT Read and Format Entries as Tree.vi"("Tree Refnum"=w283) -> ("Formatted Strings"=w284:cluster{"Name":string, "Value":string}[])  [unwired: 9 in, 1 out]
          }
        }
      }
      event "Test Tree": Value Change {
        # "Show appropriate\ncontrols"
        n177 = event-data() -> ("CtlRef"=w296:refnum<vi>, "NewVal"=w294:string)  [unwired: 1 in]
        n178 = property on="Progress" class="Clust (strict)"("Visible"=FALSE) -> ()  [unwired: 2 in, 2 out]
        n179 = call <vilib>:"WPI_UtilitiesGetTreeIOName.vi"("NewVal"=w294, "TreeControl in"=w296) -> ("I/O Name"=w297:string)  [unwired: 9 in]
        n180 = case shown="\"Camera\"" w297 {
          selector: w297 -> [_ w304 _ w322 w331 _]
          tunnel: w294 -> [_ _ w319 w321 _ w338]
          tunnel: w293 -> [_ _ _ _ _ w337]
          frame Default {
            w299 = FALSE ("Visible")
            w298 = FALSE ("Visible")
            n181 = property on="Motor" class="Clust (strict)"("Visible"=w298) -> ()  [unwired: 2 in, 2 out]
            n182 = property on="On/Off" class="Bool (strict)"("Visible"=w299) -> ()  [unwired: 2 in, 2 out]
            n183 = property on="Test Ring" class="Ring (strict)"("Visible"=w298) -> ()  [unwired: 2 in, 2 out]
            n184 = property on="Test Slider" class="Slide (strict)"("Visible"=w299) -> ()  [unwired: 2 in, 2 out]
            n185 = property on="Rev/Fwd" class="Clust (strict)"("Visible"=w299) -> ()  [unwired: 2 in, 2 out]
          }
          frame "Motor", "PWM" {
            w305 = FALSE ("Visible")
            n186 = case shown="\"Motor\", Default" w304 {
              tunnel: [1.0 ("Value") -1.0 ("Value")] -> w303
              tunnel: [255.0 ("Value") 1.0 ("Value")] -> w302
              tunnel: [128.0 ("Value") 0.0 ("Value")] -> w301
              tunnel: [64.0 ("Value") 0.5 ("Value")] -> w300
              frame "PWM" {
              }
              frame "Motor", Default {
              }
            }
            n187 = property on="On/Off" class="Bool (strict)"("Visible"=w305) -> ()  [unwired: 2 in, 2 out]
            n188 = property on="Motor" class="Clust (strict)"("Visible"=TRUE) -> ()  [unwired: 2 in, 2 out]
            n189 = property on="Test Slider" class="Slide (strict)"("Visible"=w305) -> ()  [unwired: 2 in, 2 out]
            n190 = property on="Test Ring" class="Ring (strict)"("Visible"=w305) -> ()  [unwired: 2 in, 2 out]
            n191 = property on="Rev/Fwd" class="Clust (strict)"("Visible"=w305) -> ()  [unwired: 2 in, 2 out]
            n192 = property on="Value" class="Slide (strict)"("Value"=w301, "Scale.Minimum"=w303, "Scale.Maximum"=w302, "Scale.Increment"=w300) -> ()  [unwired: 2 in, 2 out]
          }
          frame "Servo" {
            w317 = FALSE ("Visible")
            n193 = call <vilib>:"NT Read Number.vi"("Name"=w319) -> ("Numeric"=w318:dbl)  [unwired: 9 in, 1 out]
            n194 = property on="Motor" class="Clust (strict)"("Visible"=w317) -> ()  [unwired: 2 in, 2 out]
            n195 = property on="On/Off" class="Bool (strict)"("Visible"=w317) -> ()  [unwired: 2 in, 2 out]
            n196 = property on="Test Slider" class="Slide (strict)"("Visible"=TRUE, "Scale.Maximum"=170.0 ("Scale.Range:Maximum")) -> ()  [unwired: 2 in, 2 out]
            n197 = local write "Test Slider"(w318) -> ()
            n198 = property on="Test Ring" class="Ring (strict)"("Visible"=w317) -> ()  [unwired: 2 in, 2 out]
            n199 = property on="Rev/Fwd" class="Clust (strict)"("Visible"=w317) -> ()  [unwired: 2 in, 2 out]
          }
          frame "Relay", "Solenoid" {
            w320 = FALSE ("Visible")
            n200 = property on="Motor" class="Clust (strict)"("Visible"=w320) -> ()  [unwired: 2 in, 2 out]
            n201 = property on="Test Slider" class="Slide (strict)"("Visible"=w320) -> ()  [unwired: 2 in, 2 out]
            n202 = property on="Test Ring" class="Ring (strict)"("Visible"=w320) -> ()  [unwired: 2 in, 2 out]
            n203 = Search and Replace String(input string=w321, search string="/Value  **", replace string="/Direction") -> (result string=w327:string)  [unwired: 5 in, 3 out]
            n204 = call <vilib>:"NT Read String.vi"("Name"=w327) -> ("String"=w325:string)  [unwired: 9 in, 1 out]
            n205 = Equal?(x="Both directions", y=w325) -> (x = y?=w323:bool)
            n206 = property on="Rev/Fwd" class="Clust (strict)"("Visible"=w323) -> ()  [unwired: 2 in, 2 out]
            n207 = Not(x=w323) -> (.not. x?=w324:bool)
            n208 = property on="On/Off" class="Bool (strict)"("Visible"=w324, "Caption.Text"=w322) -> ()  [unwired: 2 in, 2 out]
          }
          frame "Compressor", "Digital Out" {
            w330 = FALSE ("Visible")
            # "Get direction and finish"
            n209 = property on="Motor" class="Clust (strict)"("Visible"=w330) -> ()  [unwired: 2 in, 2 out]
            n210 = property on="Rev/Fwd" class="Clust (strict)"("Visible"=FALSE) -> ()  [unwired: 2 in, 2 out]
            n211 = property on="Test Ring" class="Ring (strict)"("Visible"=w330) -> ()  [unwired: 2 in, 2 out]
            n212 = property on="Test Slider" class="Slide (strict)"("Visible"=w330) -> ()  [unwired: 2 in, 2 out]
            n213 = property on="On/Off" class="Bool (strict)"("Visible"=TRUE, "Caption.Text"=w331) -> ()  [unwired: 2 in, 2 out]
          }
          frame "Camera" {
            n214 = call <vilib>:"Get Last Path Segment.vi"("String in"=w338) -> ("String out"=w339:string)  [unwired: 10 in]
            n215 = property on="Motor" class="Clust (strict)"("Visible"=FALSE) -> ()  [unwired: 2 in, 2 out]
            n216 = case shown="\"White Balance  **\"" w339 {
              tunnel: w338 -> [w345 w354 w363 w372 w381 _ w387]
              tunnel: w337 -> [w343 w351 w360 w369 w378 _ _]
              frame "Size  **" {
                n217 = Index Array(array=w343) -> (element=w342:cluster{string[]})  [unwired: 1 in]
                n218 = call <vilib>:"NT Read String.vi"("Name"=w345) -> ("String"=w344:string)  [unwired: 9 in, 1 out]
                n219 = property on="Test Ring" class="Ring (strict)"("Visible"=TRUE) -> ()  [unwired: 2 in, 2 out]
                n220 = property on="Test Slider" class="Slide (strict)"("Visible"=FALSE) -> ()  [unwired: 2 in, 2 out]
                n221 = Unbundle(w342) -> (w340:string[])
                n222 = Match First String(2:w340, 3:w344) -> (0:w341:i32)  [unwired: 1 out]
                n223 = property on="Test Ring" class="Ring (strict)"("Value"=w341, "Strings []"=w340) -> ()  [unwired: 2 in, 2 out]
              }
              frame "White Balance  **" {
                n224 = call <vilib>:"NT Read String.vi"("Name"=w354) -> ("String"=w353:string)  [unwired: 9 in, 1 out]
                n225 = Index Array(array=w351, index=1) -> (element=w352:cluster{string[]})
                n226 = property on="Test Ring" class="Ring (strict)"("Visible"=TRUE) -> ()  [unwired: 2 in, 2 out]
                n227 = property on="Test Slider" class="Slide (strict)"("Visible"=FALSE) -> ()  [unwired: 2 in, 2 out]
                n228 = Unbundle(w352) -> (w349:string[])
                n229 = Match First String(2:w349, 3:w353) -> (0:w348:i32)  [unwired: 1 out]
                n230 = property on="Test Ring" class="Ring (strict)"("Value"=w348, "Strings []"=w349) -> ()  [unwired: 2 in, 2 out]
              }
              frame "Exposure  **" {
                n231 = call <vilib>:"NT Read String.vi"("Name"=w363) -> ("String"=w362:string)  [unwired: 9 in, 1 out]
                n232 = Index Array(array=w360, index=2) -> (element=w361:cluster{string[]})
                n233 = property on="Test Ring" class="Ring (strict)"("Visible"=TRUE) -> ()  [unwired: 2 in, 2 out]
                n234 = property on="Test Slider" class="Slide (strict)"("Visible"=FALSE) -> ()  [unwired: 2 in, 2 out]
                n235 = Unbundle(w361) -> (w357:string[])
                n236 = Match First String(2:w357, 3:w362) -> (0:w358:i32)  [unwired: 1 out]
                n237 = property on="Test Ring" class="Ring (strict)"("Value"=w358, "Strings []"=w357) -> ()  [unwired: 2 in, 2 out]
              }
              frame "Exposure Priority  **" {
                n238 = call <vilib>:"NT Read String.vi"("Name"=w372) -> ("String"=w371:string)  [unwired: 9 in, 1 out]
                n239 = Index Array(array=w369, index=3) -> (element=w370:cluster{string[]})
                n240 = property on="Test Ring" class="Ring (strict)"("Visible"=TRUE) -> ()  [unwired: 2 in, 2 out]
                n241 = property on="Test Slider" class="Slide (strict)"("Visible"=FALSE) -> ()  [unwired: 2 in, 2 out]
                n242 = Unbundle(w370) -> (w366:string[])
                n243 = Match First String(2:w366, 3:w371) -> (0:w367:i32)  [unwired: 1 out]
                n244 = property on="Test Ring" class="Ring (strict)"("Value"=w367, "Strings []"=w366) -> ()  [unwired: 2 in, 2 out]
              }
              frame "Color Enable  **" {
                n245 = call <vilib>:"NT Read String.vi"("Name"=w381) -> ("String"=w380:string)  [unwired: 9 in, 1 out]
                n246 = Index Array(array=w378, index=4) -> (element=w379:cluster{string[]})
                n247 = property on="Test Ring" class="Ring (strict)"("Visible"=TRUE) -> ()  [unwired: 2 in, 2 out]
                n248 = property on="Test Slider" class="Slide (strict)"("Visible"=FALSE) -> ()  [unwired: 2 in, 2 out]
                n249 = Unbundle(w379) -> (w375:string[])
                n250 = Match First String(2:w375, 3:w380) -> (0:w376:i32)  [unwired: 1 out]
                n251 = property on="Test Ring" class="Ring (strict)"("Value"=w376, "Strings []"=w375) -> ()  [unwired: 2 in, 2 out]
              }
              frame Default {
                n252 = property on="Test Slider" class="Slide (strict)"("Visible"=FALSE) -> ()  [unwired: 2 in, 2 out]
                n253 = property on="Test Ring" class="Ring (strict)"("Visible"=FALSE) -> ()  [unwired: 2 in, 2 out]
              }
              frame "Brightness  **", "Color Level  **", "Compression  **", "FPS  **", "Sharpness  **" {
                n254 = call <vilib>:"NT Read Number.vi"("Name"=w387) -> ("Numeric"=w386:dbl)  [unwired: 9 in, 1 out]
                n255 = property on="Test Ring" class="Ring (strict)"("Visible"=FALSE) -> ()  [unwired: 2 in, 2 out]
                n256 = property on="Test Slider" class="Slide (strict)"("Visible"=TRUE, "Scale.Maximum"=100.0 ("Scale.Range:Maximum")) -> ()  [unwired: 2 in, 2 out]
                n257 = local write "Test Slider"(w386) -> ()
              }
            }
            n258 = property on="Rev/Fwd" class="Clust (strict)"("Visible"=FALSE) -> ()  [unwired: 2 in, 2 out]
            n259 = property on="On/Off" class="Bool (strict)"("Visible"=FALSE) -> ()  [unwired: 2 in, 2 out]
          }
        }
      }
      event "Test Name": Mouse Enter {
        # "Populate the ring with the list of tests"
        n260 = event-data() -> ()  [unwired: 1 in, 1 out]
        n261 = call <vilib>:"NT Read String Array.vi"("Name"="TestMode/TestList") -> ("String Array"=w395:string[])  [unwired: 9 in, 1 out]
        n262 = Build Array (concatenate)("Select the test to run...", w395) -> (w394:string[])
        n263 = property on="Test Name" class="Ring (strict)"("Strings []"=w394) -> ()  [unwired: 2 in, 2 out]
      }
      event "Test Name": Value Change {
        w397 = FALSE ("Visible")
        # "Tell the robot the test name to run"
        n264 = event-data() -> ("NewVal"=w401:u16)  [unwired: 1 in]
        n265 = property on="Progress" class="Clust (strict)"("Visible"=TRUE) -> ()  [unwired: 2 in, 2 out]
        n266 = local write "Progress"(T11 {"Test Progress"=0, "Test Progress Text"=""} ("Progress")) -> ()
        n267 = property on="Motor" class="Clust (strict)"("Visible"=w397) -> ()  [unwired: 2 in, 2 out]
        n268 = property on="On/Off" class="Bool (strict)"("Visible"=w397) -> ()  [unwired: 2 in, 2 out]
        n269 = property on="Test Name" class="Ring (strict)"() -> ("Strings []"=w402:string[])  [unwired: 2 in, 2 out]
        n270 = property on="Test Ring" class="Ring (strict)"("Visible"=w397) -> ()  [unwired: 2 in, 2 out]
        n271 = property on="Test Slider" class="Slide (strict)"("Visible"=w397) -> ()  [unwired: 2 in, 2 out]
        n272 = property on="Rev/Fwd" class="Clust (strict)"("Visible"=w397) -> ()  [unwired: 2 in, 2 out]
        n273 = Index Array(array=w402, index=w401) -> (element=w400:string)
        n274 = call <vilib>:"NT Write String.vi"("String"=w400, "Name"="TestMode/TestName") -> ()  [unwired: 9 in, 1 out]
      }
      event "Listbox": Double Click {
        # "Shift clears all"
        # "Update symbols on the listbox"
        n275 = event-data() -> ("PlatMods.Shift"=w405:bool, "Row"=w407:i32)  [unwired: 1 in]
        n276 = case shown="True" w405 {
          tunnel: w407 -> [w411 _]
          tunnel: 1 -> [w410 _]
          frame False {
            n277 = property on="Listbox" class="LstBox (strict)"() -> ("Item Symbols"=w409:i32[])  [unwired: 2 in, 2 out]
            n278 = Replace Array Subset(array=w409, new element=w410, index=w411) -> (w408:i32[])
            n279 = property on="Listbox" class="LstBox (strict)"("Item Symbols"=w408) -> ()  [unwired: 2 in, 2 out]
          }
          frame True {
            w412 = 0 ("Top Row")
            n280 = property on="Listbox" class="LstBox (strict)"() -> ("Number of Rows"=w414:u32)  [unwired: 2 in, 2 out]
            n281 = Initialize Array(0, w414) -> (w413:i32[])
            n282 = property on="Listbox" class="LstBox (strict)"("Top Row"=w412, "Value"=w412, "Item Symbols"=w413) -> ()  [unwired: 2 in, 2 out]
          }
        }
      }
      event "Listbox": Key Down {
        # "Update symbols on the listbox\nLeft and right keys check and uncheck"
        n283 = event-data() -> ("VKey"=w418:T27)  [unwired: 1 in]
        n284 = case shown="\"Left\", \"Right\"" w418 {
          selector: w418 -> [w423 _]
          tunnel: eventvkey."Left" ("VKey") -> [w421 _]
          frame "Left", "Right" {
            n285 = Equal?(x=w421, y=w423) -> (x = y?=w422:bool)
            n286 = Select(t=0, s=w422, f=1) -> (s? t:f=w424:i32)
            n287 = property on="Listbox" class="LstBox (strict)"() -> ("Item Symbols"=w427:i32[])  [unwired: 2 in, 2 out]
            n288 = Replace Array Subset(array=w427, new element=w424, index="Listbox") -> (w426:i32[])
            n289 = property on="Listbox" class="LstBox (strict)"("Item Symbols"=w426) -> ()  [unwired: 2 in, 2 out]
          }
          frame Default {
          }
        }
      }
      event "DB Camera Config": Value Change {
        # "Show or hide the cluster of controls, store in ini file"
        n290 = event-data() -> ("NewVal"=w431:bool)  [unwired: 1 in]
        n291 = case shown="False" w431 {
          tunnel: w430 -> [w440 _]
          tunnel: [w433 w451] -> w429
          tunnel: w428 -> [w432 w451]
          frame False {
            w447 = "Camera"
            w450 = FALSE ("Visible")
            n292 = property on="Camera Settings" class="Clust (strict)"("Visible"=w450) -> ()  [unwired: 2 in, 2 out]
            n293 = local write "DB Camera Config"(w450) -> ()
            n294 = local read "Camera Settings"() -> (w439:T2)
            n295 = Index Array(array=w440) -> (element=w443:cluster{string[]})  [unwired: 1 in]
            n296 = Unbundle(w443) -> (w442:string[])
            n297 = Unbundle(w439) -> ("Frame Rate"=w438:i32, "Compression"=w437:i32, "Size"=w441:u16)
            n298 = Index Array(array=w442, index=w441) -> (element=w436:string)
            n299 = call-poly <vilib>:"Write Key.vi"("section"=w447, "value"=w436, "key"="Size", "refnum"=w432) -> ("refnum out"=w449:T15)  [unwired: 2 in, 5 out]
            n300 = call-poly <vilib>:"Write Key.vi"("section"=w447, "value"=w438, "key"="FrameRate", "refnum"=w449) -> ("refnum out"=w448:T15)  [unwired: 1 in, 6 out]
            n301 = call-poly <vilib>:"Write Key.vi"("section"=w447, "value"=w437, "key"="Compression", "refnum"=w448) -> ("refnum out"=w434:T15)  [unwired: 1 in, 6 out]
            n302 = call <vilib>:"Close Config Data.vi"("refnum"=w434) -> ("file path"=w435:path)  [unwired: 2 in, 8 out]
            n303 = call <vilib>:"Open Config Data.vi"("configuration file path"=w435) -> ("refnum"=w433:T15)  [unwired: 8 in, 2 out]
          }
          frame True {
            n304 = property on="Camera Settings" class="Clust (strict)"("Visible"=TRUE) -> ()  [unwired: 2 in, 2 out]
          }
        }
      }
      event "Camera Settings": Value Change {
        # "Update summary string when any elements of DB camera change"
        n305 = event-data() -> ("NewVal"=w464:T2)  [unwired: 1 in]
        n306 = Index Array(array=w460) -> (element=w459:cluster{string[]})  [unwired: 1 in]
        n307 = Unbundle(w459) -> (w458:string[])
        n308 = Unbundle(w464) -> ("Frame Rate"=w455:i32, "Compression"=w454:i32, "Size"=w457:u16)
        n309 = Index Array(array=w458, index=w457) -> (element=w456:string)
        n310 = Format Into String(format string="%s   %dfps   %d%%", w456, w455, w454) -> (resulting string=w461:string)  [unwired: 2 in, 1 out]
        n311 = Build Array(w461) -> (w462:string[])
        n312 = property on="DB Camera Config" class="Bool (strict)"("Strings [4]"=w462) -> ()  [unwired: 2 in, 2 out]
      }
      event "Motor.Enable": Value Change {
        # "When the test mode otor enable helper is set, update that\ntree row item's value"
        n313 = event-data() -> ("NewVal"=w470:bool)  [unwired: 1 in]
        n314 = Unbundle("Motor") -> ("Value"=w469:dbl)  [unwired: 1 out]
        n315 = Select(t=w469, s=w470, f=0.0) -> (s? t:f=w467:dbl)
        n316 = call <vilib>:"NT Write Number.vi"("Numeric"=w467, "Name"=w466) -> ()  [unwired: 9 in, 1 out]
      }
      event "Test Slider": Value Change {
        # "When the test mode slider helper is set, update that\ntree row item's value"
        n317 = event-data() -> ("NewVal"=w473:dbl)  [unwired: 1 in]
        n318 = call <vilib>:"NT Write Number.vi"("Numeric"=w473, "Name"=w474) -> ()  [unwired: 9 in, 1 out]
      }
      event "On/Off": Value Change {
        # "When the test mode on/off helper value is set, update that\ntree row item's value"
        n319 = event-data() -> ("NewVal"=w478:bool)  [unwired: 1 in]
        n320 = Boolean To (0,1)(Boolean=w478) -> (0, 1=w477:i16)
        n321 = call <vilib>:"NT Write Number.vi"("Numeric"=w477, "Name"=w476) -> ()  [unwired: 9 in, 1 out]
      }
      event "Rev/Fwd": Value Change {
        # "When the test mode helper value for relays is set, update that\ntree row item's value"
        n322 = event-data() -> ("NewVal.Forward"=w486:bool, "NewVal.Reverse"=w485:bool)  [unwired: 1 in]
        n323 = Boolean To (0,1)(Boolean=w485) -> (0, 1=w484:i16)
        n324 = Boolean To (0,1)(Boolean=w486) -> (0, 1=w482:i16)
        n325 = Negate(x=w484) -> (-x=w483:i16)
        n326 = Add(x=w482, y=w483) -> (x+y=w481:i16)
        n327 = call <vilib>:"NT Write Number.vi"("Numeric"=w481, "Name"=w480) -> ()  [unwired: 9 in, 1 out]
      }
      event "Test Ring": Value Change {
        # "When a test mode helper value is selected from the ring,\nset the tree item's variable to the string value"
        n328 = event-data() -> ("NewVal"=w490:u16)  [unwired: 1 in]
        n329 = property on="Test Ring" class="Ring (strict)"() -> ("Strings []"=w491:string[])  [unwired: 2 in, 2 out]
        n330 = Index Array(array=w491, index=w490) -> (element=w489:string)
        n331 = call <vilib>:"NT Write String.vi"("String"=w489, "Name"=w488) -> ()  [unwired: 9 in, 1 out]
      }
      event "Rec Mode": Value Change {
        # "Update globals for recording mode and path to read log from.\nClear when logging and let NetworkTables set path for vision to\nuse."
        n332 = event-data() -> ("NewVal"=w501:enum32{"Stop", "Record", "Playback"})  [unwired: 1 in]
        n333 = global write "WPI_DashboardLogging Global.vi" "Logging Filename"(path "") -> ()
        n334 = global write "WPI_DashboardLogging Global.vi" "Recording"(w501) -> ()
        n335 = call <vilib>:"WPI_DashboardNT Log FieldName Cache.vi"("Operation"=enum16{"Lookup/Add", "Index", "Clear"}."Clear") -> ()  [unwired: 8 in, 3 out]
        n336 = case shown="\"Playback\"" w501 {
          tunnel: w500 -> [_ w503 w511]
          tunnel: [_ _ w510] -> w497
          tunnel: [_ _ w509] -> _
          tunnel: w495 -> [_ _ w507]
          tunnel: cluster{i32, i32} {-250, 170} -> [_ _ w506]
          tunnel: [_ _ T28 {"Image Size"=TRUE, "Image Type"=TRUE, "Pixel Value"=TRUE, "ROI Information"=TRUE, "Zoom Factor"=FALSE} ("Image Information Shown:All Elements")] -> w493
          tunnel: [_ _ TRUE ("Zoom Factor")] -> w492
          frame Default {
          }
          frame "Stop", "Record" {
            # "Place Window too"
            n337 = invoke class="VI" method="FP.Close"(reference=w503) -> (reference out=w502:refnum<vi>)  [unwired: 2 in, 2 out]
            n338 = invoke class="VI" method="Abort VI"(reference=w502) -> ()  [unwired: 2 in, 3 out]
          }
          frame "Playback" {
            n339 = call "Open Playback Panel.vi"("Offset"=w506, "DB VI Ref"=w507, "Playback in"=w511) -> ("Playback out"=w508:refnum<vi>)  [unwired: 8 in]
            n340 = register-events(w508) -> (reference out=w510:refnum<event-registration>, error out=w509:errorcluster)  [unwired: 2 in]
          }
        }
        n341 = property on="Camera Image" class="ImageControl"("Image Information Shown"=w493, "Image Information Visible"=w492) -> ()  [unwired: 2 in, 2 out]
      }
      event Panel Close {
        w512 = enum32{"Stop", "Record", "Playback"}."Stop" ("Rec Mode")
        # "Playback window has been closed, abort"
        n342 = event-data() -> ()  [unwired: 1 in, 4 out]
        n343 = local write "Rec Mode"(w512) -> ()
        n344 = global write "WPI_DashboardLogging Global.vi" "Recording"(w512) -> ()
      }
      event Panel Close {
        # "Abort playback window and ourself"
        n345 = event-data() -> ()  [unwired: 1 in, 4 out]
        n346 = invoke class="VI" method="FP.Close"(reference=w517) -> (reference out=w516:refnum<vi>)  [unwired: 2 in, 2 out]
        n347 = invoke class="VI" method="Abort VI"(reference=w516) -> (error out=w515:errorcluster)  [unwired: 2 in, 2 out]
        n348 = invoke class="VI" method="Abort VI"(error in=w515) -> ()  [unwired: 2 in, 3 out]
      }
      event "Vision": Value Change {
        # "Enable/Disable Compression slider.\nHW USB is hard-coded into the camera"
        n349 = event-data() -> ("NewVal"=w523:u16)  [unwired: 1 in]
        n350 = Equal?(x=w523, y=u32 2 ("milliseconds to wait")) -> (x = y?=w521:bool)
        n351 = Select(t=T29."Disabled and Grayed Out" ("Disabled"), s=w521, f=T29."Enabled" ("Disabled")) -> (s? t:f=w518:T29)
        n352 = property on="Compression" class="Slide (strict)"("DisabledEnum"=w518) -> ()  [unwired: 2 in, 2 out]
      }
    }
  }
